vi "Get DDGIOC Period.vi"(11 "period":cluster{}) -> (2 "function return":u32, 3 "period out":cluster{})   [LabVIEW 2018, in "Copy of Andor SDK.lvlib"]
doc: "EXPNETTYPE unsigned int WINAPI GetDDGIOCPeriod(at_u64 * period);"
uses:
  Copy of Andor SDK.lvlib
  <userlib>/Andor SDK/ATMCD32D.dll
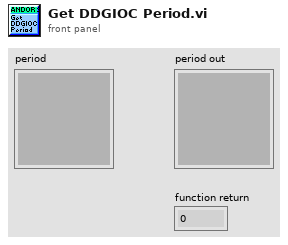
[diagram p1: front panel]
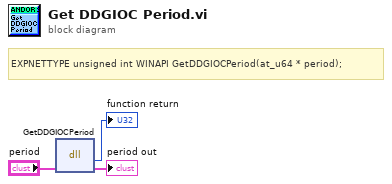
[diagram p0: block diagram]
diagram:
  # "EXPNETTYPE unsigned int WINAPI GetDDGIOCPeriod(at_u64 * period);"
  n1 = dll-call lib="C:/Program Files (x86)/National Instruments/LabVIEW 2018/user.lib/Andor SDK/ATMCD32D.*" fn="GetDDGIOCPeriod"("period"="period") -> (→"function return":u32, "period"=→"period out":cluster{})  [unwired: 3 in, 2 out]
